vi "SQLite Add Category Test.vi"(7 "Test DB Set Up Command":string, 8 "Error In (no error)":errorcluster, 11 "SQLite DB Operator In":refnum<class "SQLite DB Operator.lvclass">) -> (0 "Error Out":errorcluster, 3 "SQLite DB OperatorOut":refnum<class "SQLite DB Operator.lvclass">)   [LabVIEW 2023]
uses:
  Clasess/SQLite DB Operator/SQLite DB Operator.lvclass
  Clasess/DB Records/Expenses Tracker Category/Public/Ctrls/Category.ctl
  Clasess/DB Records/Expenses Tracker Category/Expenses Tracker Category.lvclass
  H:/Desktop/LabVIEW/LabView Repo/Expenses-Tracker-DB-Operator/Interfaces/Expenses Tracker Record/Expenses Tracker Record.lvclass
  <vilib>/drjdpowell/SQLite Library/SQL Connection/Execute SQL (1D Cluster).vi
  <vilib>/addons/_JKI Toolkits/Caraya/classes/Test/Test.lvclass
  <vilib>/drjdpowell/SQLite Library/SQLite.lvlib
  <vilib>/drjdpowell/SQLite Library/SQL Connection/Connection.lvclass
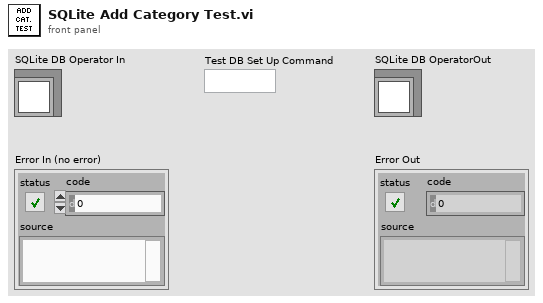
[diagram p1: front panel]
types:
  T1 = typedef "Expenses Tracker Category.lvclass/Category.ctl" = cluster{"ID":u32, "Name":string}
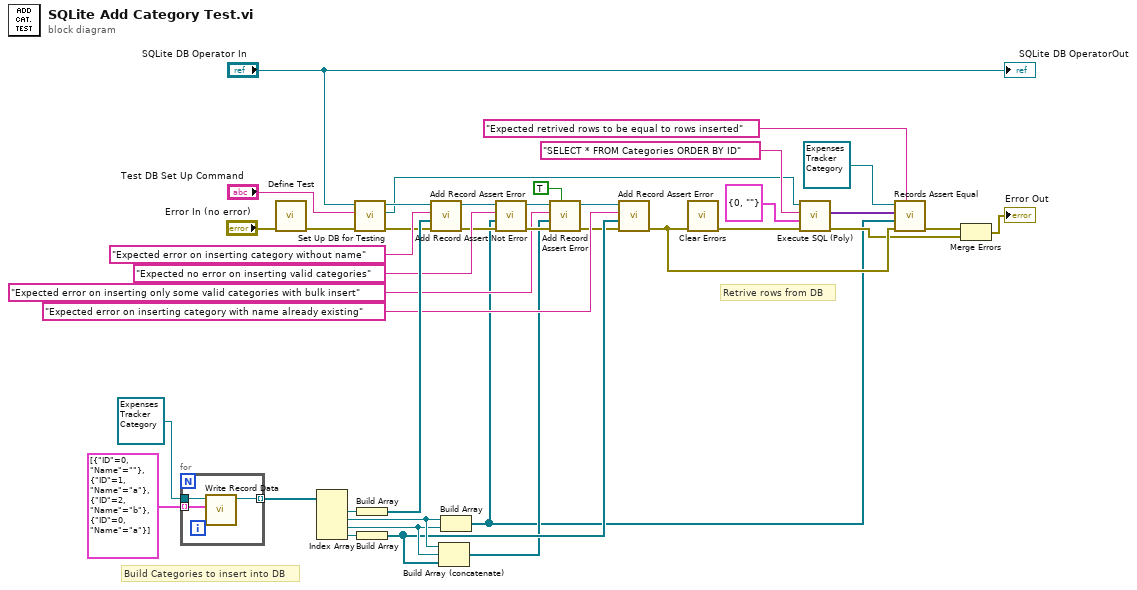
[diagram p0: block diagram]
diagram:
  # "Retrive rows from DB"
  # "Build Categories to insert into DB"
  n1 = for {
    tunnel: T1[] [{"ID"=0, "Name"=""}, {"ID"=1, "Name"="a"}, {"ID"=2, "Name"="b"}, {"ID"=0, "Name"="a"}] ("Array") -> [w42] mode=indexing
    tunnel: refnum<class "Expenses Tracker Category.lvclass"> refnum ("Expenses Tracker Category") -> [w41]
    tunnel: [w40] -> w36 mode=indexing
    n2 = call-dynamic "Write Record Data.vi"("Record"=w42, "Expenses Tracker Category In"=w41) -> ("Expenses Tracker Category Out"=w40:refnum<class "Expenses Tracker Category.lvclass">)  [unwired: 8 in, 1 out]
  }
  n3 = call <vilib>:"Define Test.vi"("error in (no error)"="Error In (no error)") -> ("error out"=w24:errorcluster)  [unwired: 9 in, 1 out]
  n4 = Index Array(array=w36) -> (element #1=w35:refnum<class "Expenses Tracker Category.lvclass">, element #2=w11:refnum<class "Expenses Tracker Category.lvclass">, element #3=w10:refnum<class "Expenses Tracker Category.lvclass">, element #4=w33:refnum<class "Expenses Tracker Category.lvclass">)  [unwired: 4 in]
  n5 = call "Set Up DB for Testing.vi"("Error In (no error)"=w24, "Test DB Set Up Command"="Test DB Set Up Command", "SQLite DB Operator In"="SQLite DB Operator In") -> ("Error Out"=w23:errorcluster, "SQLite Connection"=w26:refnum<class "Connection.lvclass">, "SQLite DB Operator Out"=w28:refnum<class "SQLite DB Operator.lvclass">)  [unwired: 6 in]
  n6 = Build Array(w35) -> (w34:refnum<class "Expenses Tracker Category.lvclass">[])
  n7 = Build Array(w33) -> (w9:refnum<class "Expenses Tracker Category.lvclass">[])
  n8 = call "Add Record Assert Error.vi"("Error In"=w23, "Records"=w34, "Assertion Label"="Expected error on inserting category without name" ("Label (VI Title)"), "SQLite DB Operator In"=w28) -> ("Error Out"=w20:errorcluster, "SQLite DB Operator Out"=w22:refnum<class "SQLite DB Operator.lvclass">)  [unwired: 6 in]
  n9 = Build Array (concatenate)(w11, w10, w9) -> (w3:refnum<class "Expenses Tracker Category.lvclass">[])
  n10 = Build Array(w11, w10) -> (w2:refnum<class "Expenses Tracker Category.lvclass">[])
  n11 = call "Add Record Assert Not Error.vi"("Error In"=w20, "Records"=w2, "Assertion Label"="Expected no error on inserting valid categories" ("Label (VI Title)"), "SQLite DB Operator In"=w22) -> ("Error Out"=w8:errorcluster, "SQLite DB Operator Out"=w7:refnum<class "SQLite DB Operator.lvclass">)  [unwired: 6 in]
  n12 = call "Add Record Assert Error.vi"("Bulk Insert?"=TRUE, "Error In"=w8, "Records"=w3, "Assertion Label"="Expected error on inserting only some valid categories with bulk insert" ("Label (VI Title)"), "SQLite DB Operator In"=w7) -> ("Error Out"=w6:errorcluster, "SQLite DB Operator Out"=w5:refnum<class "SQLite DB Operator.lvclass">)  [unwired: 5 in]
  n13 = call "Add Record Assert Error.vi"("Error In"=w6, "Records"=w9, "Assertion Label"="Expected error on inserting category with name already existing" ("Label (VI Title)"), "SQLite DB Operator In"=w5) -> ("Error Out"=w16:errorcluster)  [unwired: 6 in, 1 out]
  n14 = call <vilib>:"Clear Errors.vi"("error in (no error)"=w16) -> ("error out"=w17:errorcluster)  [unwired: 5 in, 1 out]
  n15 = call-poly <vilib>:"Execute SQL (Poly).vi"("error in (no error)"=w17, "Cluster (or Array of Clusters)"=T1 {"ID"=0, "Name"=""} ("Category"), "SQL"="SELECT * FROM Categories ORDER BY ID", "SQLite Connection in"=w26) -> ("error out"=w13:errorcluster, "Result Set (Array of Clusters)"=w31:variant[])  [unwired: 5 in, 1 out]
  n16 = call "Records Assert Equal.vi"("Assertion Label"="Expected retrived rows to be equal to rows inserted" ("Label (VI Title)"), "Error In"=w16, "Correct Records"=w2, "Typedef Records"=w31, "Expenses Tracker Record In"=refnum<class "Expenses Tracker Category.lvclass"> refnum ("Expenses Tracker Category")) -> ("Error Out"=w29:errorcluster)  [unwired: 6 in]
  n17 = Merge Errors(w29, w13) -> (→"Error Out":errorcluster)
  "SQLite DB OperatorOut" <- "SQLite DB Operator In"
